vi "JSON reading_RC.vi"(8 "error in":errorcluster, 10 "Override file path":path=path "C:/Users/veenaj/Desktop/ZenGage V1.3/Configuration file/Rack Controller Parameters Override.json", 11 "Default file path":path=path "C:/Users/veenaj/Desktop/ZenGage V1.3/Configuration file/Rack Controller Parameters Default.json") -> (0 "error out":errorcluster, 3 "Output Merged Cluster":variant=variant(cluster{"SpecificationVersion":string, "CompatibleSoftwareVersions":variant[], "RackControllerParameters":variant[]} {"SpecificationVersion"="1", "CompatibleSoftwareVersions"=[variant(string "1.0")], "RackControllerParameters"=[variant(cluster{"RackId":u64, "FrontPanelOpen":bool, "PartsList":variant[]} {"RackId"=0, "FrontPanelOpen"=FALSE, "PartsList"=[variant(cluster{"Name":string, "Measurements":variant[], "UnloadPositionCounts":cluster{"Fail":u64, "ReelEnd":u64, "ProductionEnd":u64}} {"Name"="HSG 250F (PS03)", "Measurements"=[variant(cluster{"MeasurementId":u64, "Name":string, "ControlLimitsViolationThreshold":cluster{"AllowableFails":u64, "WindowSize":u64}, "SpecificationLimitViolationThreshold":cluster{"AllowableFails":u64, "WindowSize":u64}} {"MeasurementId"=0, "Name"="A", "ControlLimitsViolationThreshold"={"AllowableFails"=1, "WindowSize"=1}, "SpecificationLimitViolationThreshold"={"AllowableFails"=1, "WindowSize"=1}}), variant(cluster{"MeasurementId":u64, "Name":string, "ControlLimitsViolationThreshold":cluster{"AllowableFails":u64, "WindowSize":u64}, "SpecificationLimitViolationThreshold":cluster{"AllowableFails":u64, "WindowSize":u64}} {"MeasurementId"=2, "Name"="B", "ControlLimitsViolationThreshold"={"AllowableFails"=1, "WindowSize"=1}, "SpecificationLimitViolationThreshold"={"AllowableFails"=1, "WindowSize"=1}}), variant(cluster{"MeasurementId":u64, "Name":string, "ControlLimitsViolationThreshold":cluster{"AllowableFails":u64, "WindowSize":u64}, "SpecificationLimitViolationThreshold":cluster{"AllowableFails":u64, "WindowSize":u64}} {"MeasurementId"=3, "Name"="C", "ControlLimitsViolationThreshold"={"AllowableFails"=1, "WindowSize"=1}, "SpecificationLimitViolationThreshold"={"AllowableFails"=1, "WindowSize"=1}}), variant(cluster{"MeasurementId":u64, "Name":string, "ControlLimitsViolationThreshold":cluster{"AllowableFails":u64, "WindowSize":u64}, "SpecificationLimitViolationThreshold":cluster{"AllowableFails":u64, "WindowSize":u64}} {"MeasurementId"=4, "Name"="D", "ControlLimitsViolationThreshold"={"AllowableFails"=1, "WindowSize"=1}, "SpecificationLimitViolationThreshold"={"AllowableFails"=1, "WindowSize"=1}})], "UnloadPositionCounts"={"Fail"=10, "ReelEnd"=10, "ProductionEnd"=10}})]})]}))   [LabVIEW 2019, in "Rack Controller.lvclass"]
uses:
  Rack Controller.lvclass
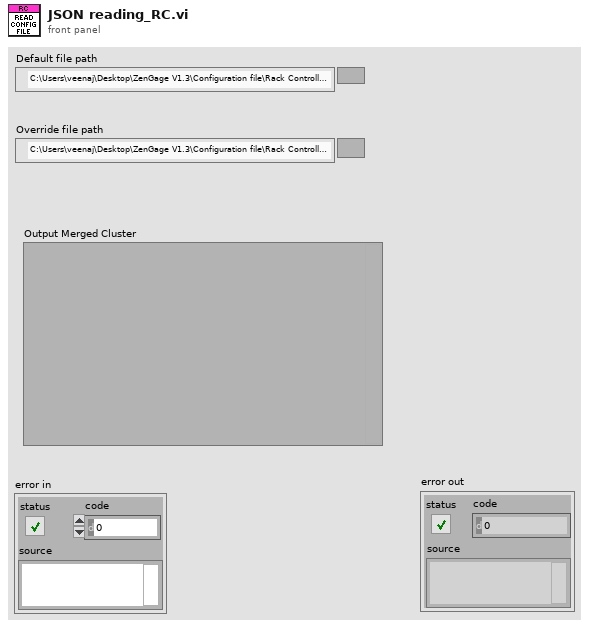
[diagram p1: front panel]
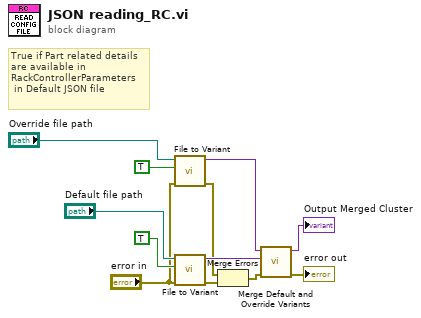
[diagram p0: block diagram]
diagram:
  # "True if Part related details\nare available in\nRackControllerParameters\n in Default JSON file"
  n1 = call <vilib>:"File to Variant.vi"("JSON FilePath"="Override file path", "Remove Comments?"=TRUE, "error in (no error)"="error in") -> ("JSON Variant"=w7:variant, "error out"=w5:errorcluster)  [unwired: 5 in, 1 out]
  n2 = call <vilib>:"File to Variant.vi"("JSON FilePath"="Default file path", "Remove Comments?"=TRUE, "error in (no error)"="error in") -> ("JSON Variant"=w6:variant, "error out"=w4:errorcluster)  [unwired: 5 in, 1 out]
  n3 = Merge Errors(w5, w4) -> (w3:errorcluster)
  n4 = call <vilib>:"Merge Default and Override Variants.vi"("error in (no error)"=w3, "Default VCluster"=w6, "Override VCluster"=w7) -> ("error out"=→"error out":errorcluster, "Output Merged Cluster"=→"Output Merged Cluster":variant)  [unwired: 7 in]
